vi "svse_StopFGV.vi"(7 "Reset (F)":bool, 10 "error in":errorcluster, 11 "User stop? (F)":bool) -> (2 "error out":errorcluster, 3 "Stop?":bool)   [LabVIEW 2011]
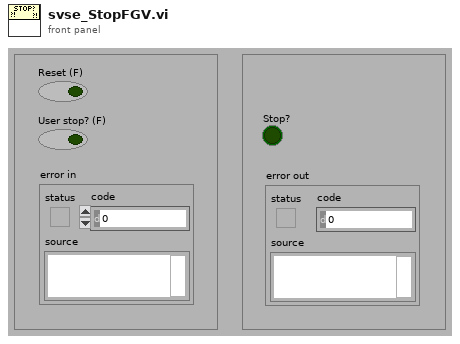
[diagram p1: front panel]
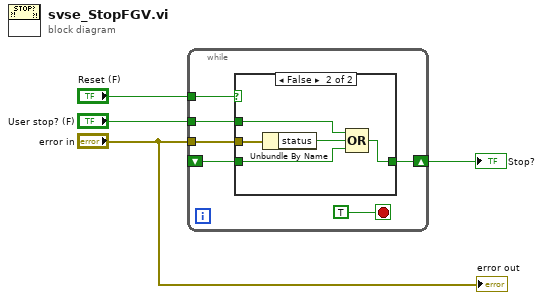
[diagram p0: block diagram]
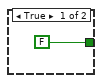
[diagram p2: hidden frame]
diagram:
  n1 = while {
    tunnel: "error in" -> [w10]
    shift-right: [w9] -> w4
    shift-left: _ -> [w8]
    tunnel: "Reset (F)" -> [w7]
    tunnel: "User stop? (F)" -> [w5]
    stop <- TRUE stop-if-true
    n2 = case shown="False" w7 {
      tunnel: w10 -> [_ w16]
      tunnel: [FALSE w13] -> w9
      tunnel: w8 -> [_ w15]
      tunnel: w5 -> [_ w12]
      frame True {
      }
      frame False {
        n3 = Unbundle By Name(w16) -> ("status"=w14:bool)
        n4 = Compound Arithmetic op=OR(w12, w14, w15) -> (w13:bool)
      }
    }
  }
  "Stop?" <- w4
  "error out" <- "error in"
